vi "lab session 7.2.vi"() -> ()   [LabVIEW 2020]
uses:
  <vilib>/numeric/Random Number (Range) U64.vi
  <vilib>/numeric/sub_Random U32.vi
panel:
  in  "Delat time in ms":dbl
  out "row":dbl
  out "column":dbl
  in  "sq matirx size":dbl
  out "Array":u64[][](array[numeric])
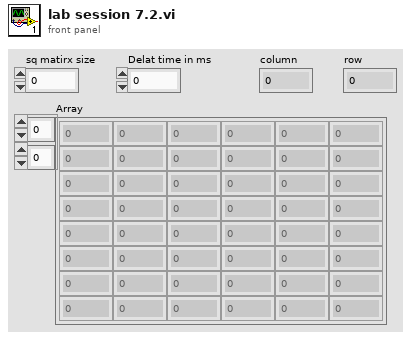
[diagram p1: front panel]
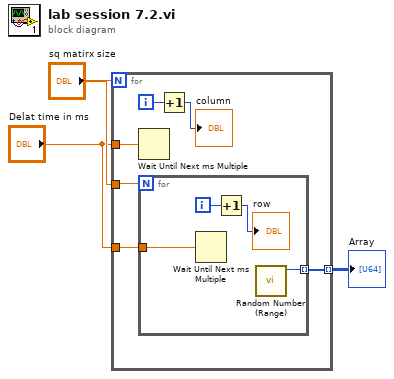
[diagram p0: block diagram]
diagram:
  n1 = for {
    N: "sq matirx size" -> [_]
    tunnel: [w9] -> w3 mode=indexing
    tunnel: "sq matirx size" -> [w8]
    tunnel: "Delat time in ms" -> [w7]
    tunnel: "Delat time in ms" -> [w6]
    i -> [w5]
    n2 = Wait Until Next ms Multiple(millisecond multiple=w7) -> ()  [unwired: 1 out]
    n3 = for {
      N: w8 -> [_]
      tunnel: [w13] -> w9 mode=indexing
      tunnel: w6 -> [w12]
      i -> [w11]
      n4 = Wait Until Next ms Multiple(millisecond multiple=w12) -> ()  [unwired: 1 out]
      n5 = Increment(x=w11) -> (x+1=→"row":i32)
      n6 = call-poly <vilib>:"Random Number (Range).vi"() -> ("number"=w13:u64)  [unwired: 11 in]
    }
    n7 = Increment(x=w5) -> (x+1=→"column":i32)
  }
  "Array" <- w3
